vi "dfd_Validate Coef Setting Pair.vi"(7 "coef b/v wl":i16, 8 "error in (no error)":errorcluster, 11 "coef a/k wl":i16) -> (0 "error out":errorcluster, 3 "a/k selector":bool, 5 "b/v selector":bool)   [LabVIEW 2017, in "NI_DigFilter_FXP.lvlib"]
uses:
  <vilib>/addons/Digital Filter Design/NI_DigFilter_FXP.lvlib
  <vilib>/addons/Digital Filter Design/_Misc.llb/dfd_Error Handlers (Single).vi
  <vilib>/addons/Digital Filter Design/NI_DigFilterLicensed.lvlib
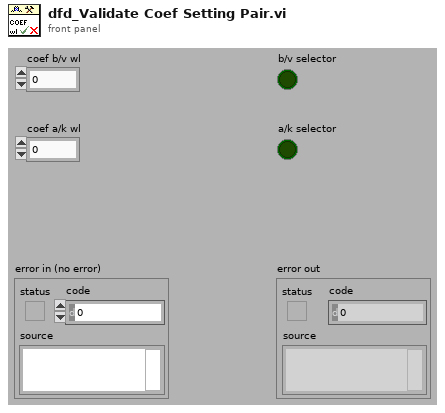
[diagram p1: front panel]
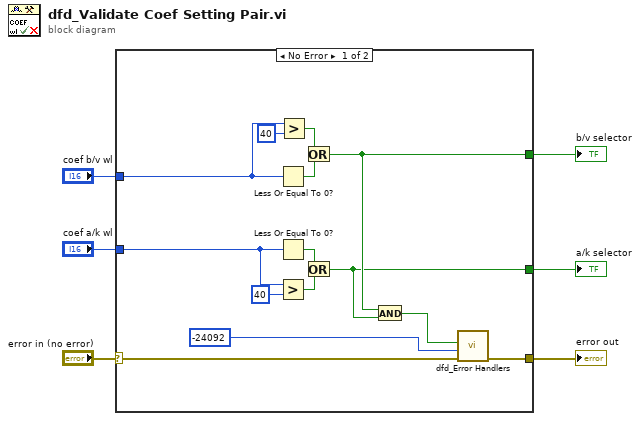
[diagram p0: block diagram]
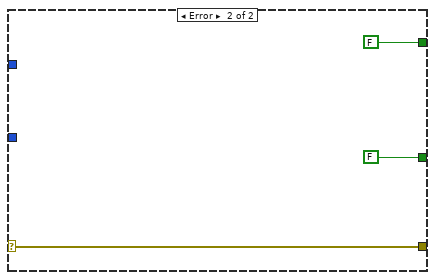
[diagram p2: hidden frame]
diagram:
  n1 = case shown="No Error" "error in (no error)" {
    selector: "error in (no error)" -> [w12 w23]
    tunnel: [w11 w23] -> w5
    tunnel: "coef b/v wl" -> [w15 _]
    tunnel: "coef a/k wl" -> [w14 _]
    tunnel: [w8 FALSE] -> w2
    tunnel: [w7 FALSE] -> w1
    frame No Error {
      n2 = Less Or Equal To 0?(x=w15) -> (x <= 0?=w18:bool)
      n3 = Less Or Equal To 0?(x=w14) -> (x <= 0?=w16:bool)
      n4 = Greater?(x=w14, y=i16 40) -> (0:w13:bool)
      n5 = Greater?(x=w15, y=i16 40) -> (0:w19:bool)
      n6 = Or(x=w19, y=w18) -> (x .or. y?=w8:bool)
      n7 = Or(x=w16, y=w13) -> (x .or. y?=w7:bool)
      n8 = And(x=w8, y=w7) -> (x .and. y?=w10:bool)
      n9 = call-poly <vilib>:"dfd_Error Handlers.vi"("error in (no error)"=w12, "error code"=-24092 ("ERR_INVALID_COEF_WL"), "condition failed?"=w10) -> ("error out"=w11:errorcluster)  [unwired: 8 out]
    }
    frame Error {
    }
  }
  "a/k selector" <- w1
  "error out" <- w5
  "b/v selector" <- w2
